vi "modbus-conver.vi"(6 "Reg":dbl, 8 "error in (no error)":errorcluster, 9 "Scale Min range":dbl, 10 "Scale Max Range":dbl, 11 "object in":refnum<class "Type-T-Thermocouple.lvclass">) -> (0 "error out":errorcluster, 2 "output":dbl, 3 "object out":refnum<class "Type-T-Thermocouple.lvclass">)   [LabVIEW 2016, in "Type-T-Thermocouple.lvclass"]
doc: "formula to convert adam modbus to real"
uses:
  Type-T-Thermocouple.lvclass
  Modbus-Instr_class/Modbus-Instr.lvclass
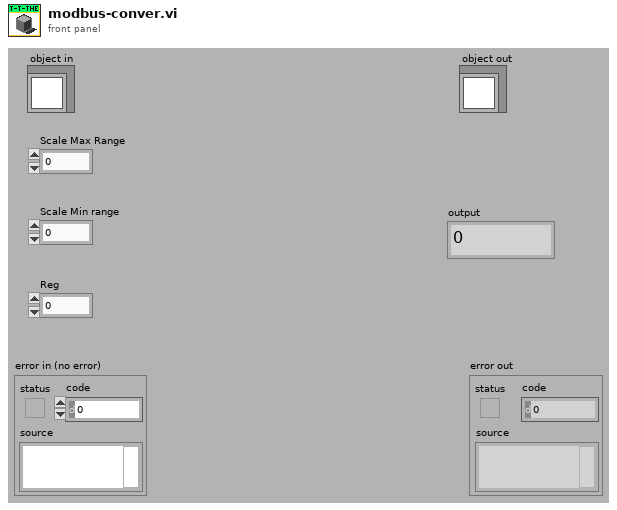
[diagram p1: front panel]
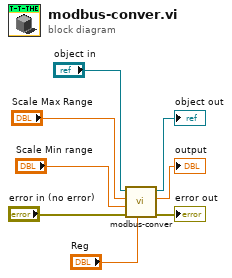
[diagram p0: block diagram]
diagram:
  n1 = call-parent "modbus-conver.vi"("Reg"="Reg", "error in (no error)"="error in (no error)", "Scale Min range"="Scale Min range", "Scale Max Range"="Scale Max Range", "object in"="object in") -> ("error out"=→"error out":errorcluster, "output"=→"output":dbl, "object out"=→"object out":refnum<class "Type-T-Thermocouple.lvclass">)  [unwired: 4 in]
